vi "code_template.vi"(8 "ERRORIN":errorcluster, 10 "DATA":variant, 11 "CMD":string) -> (0 "ERROROUT":errorcluster, 3 "MSG":cluster{"cmd":string, "data":variant})   [LabVIEW 2025]
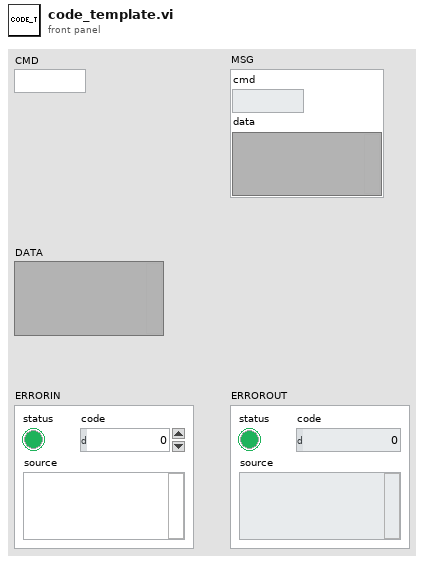
[diagram p1: front panel]
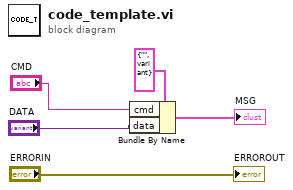
[diagram p0: block diagram]
diagram:
  n1 = Bundle By Name(cluster=cluster{"cmd":string, "data":variant} {"cmd"="", "data"=variant} ("element"), "cmd"="CMD", "data"="DATA") -> (→"MSG":cluster{"cmd":string, "data":variant})
  "ERROROUT" <- "ERRORIN"
